vi "test-unscented-kalman-filter-3.vi"() -> (3 "Test good":bool)   [LabVIEW 2019]
uses:
  <vilib>/Analysis/Matrix/Datatypes/RealMatrix.ctl
  <vilib>/Rock Robotics/WPI/ThirdParty/JAS_Junk/TrajLib/MatBuilder_Create.vi
  <vilib>/Rock Robotics/WPI/ThirdParty/JAS_Junk/TrajLib/CallbackHelp_MatrixMinus.vi
  <vilib>/Rock Robotics/WPI/ThirdParty/JAS_Junk/TrajLib/CallbackHelp_MatrixMult_CoerceSizeB.vi
  <vilib>/Rock Robotics/WPI/ThirdParty/JAS_Junk/TrajLib/Trajectory_Library.lvlib
  <vilib>/Analysis/Matrix/NI_Matrix.lvlib
panel:
  out "P Passed":bool
  out "X Passed":bool
  out "P":T1
  out "X":T1
  out "Error":bool
  # "assertTrue(VecBuilder.fill(-0.9, 1, -0.9, 1).isEqual(ret.getFirst(), 1E-5));"
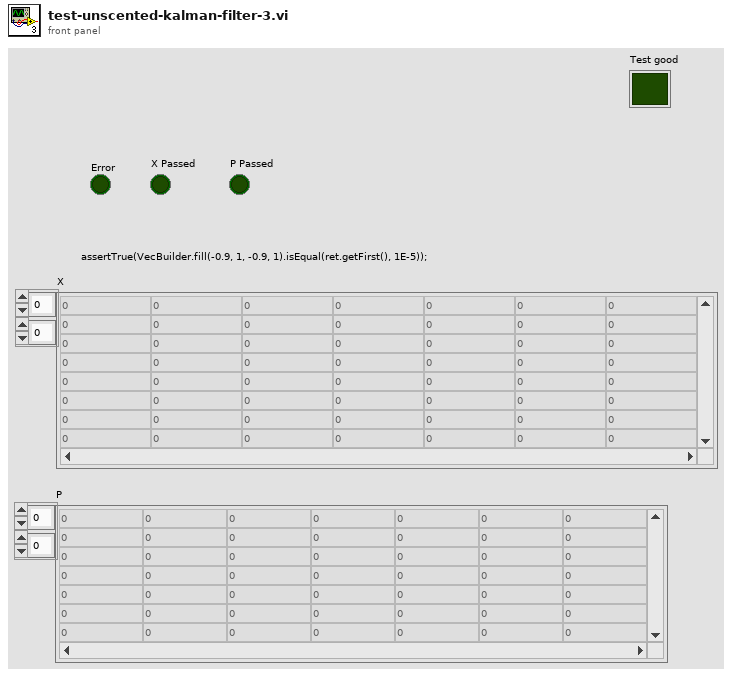
[diagram p1: front panel]
types:
  T1 = typedef "NI_Matrix.lvlib/RealMatrix.ctl" = dbl[][]
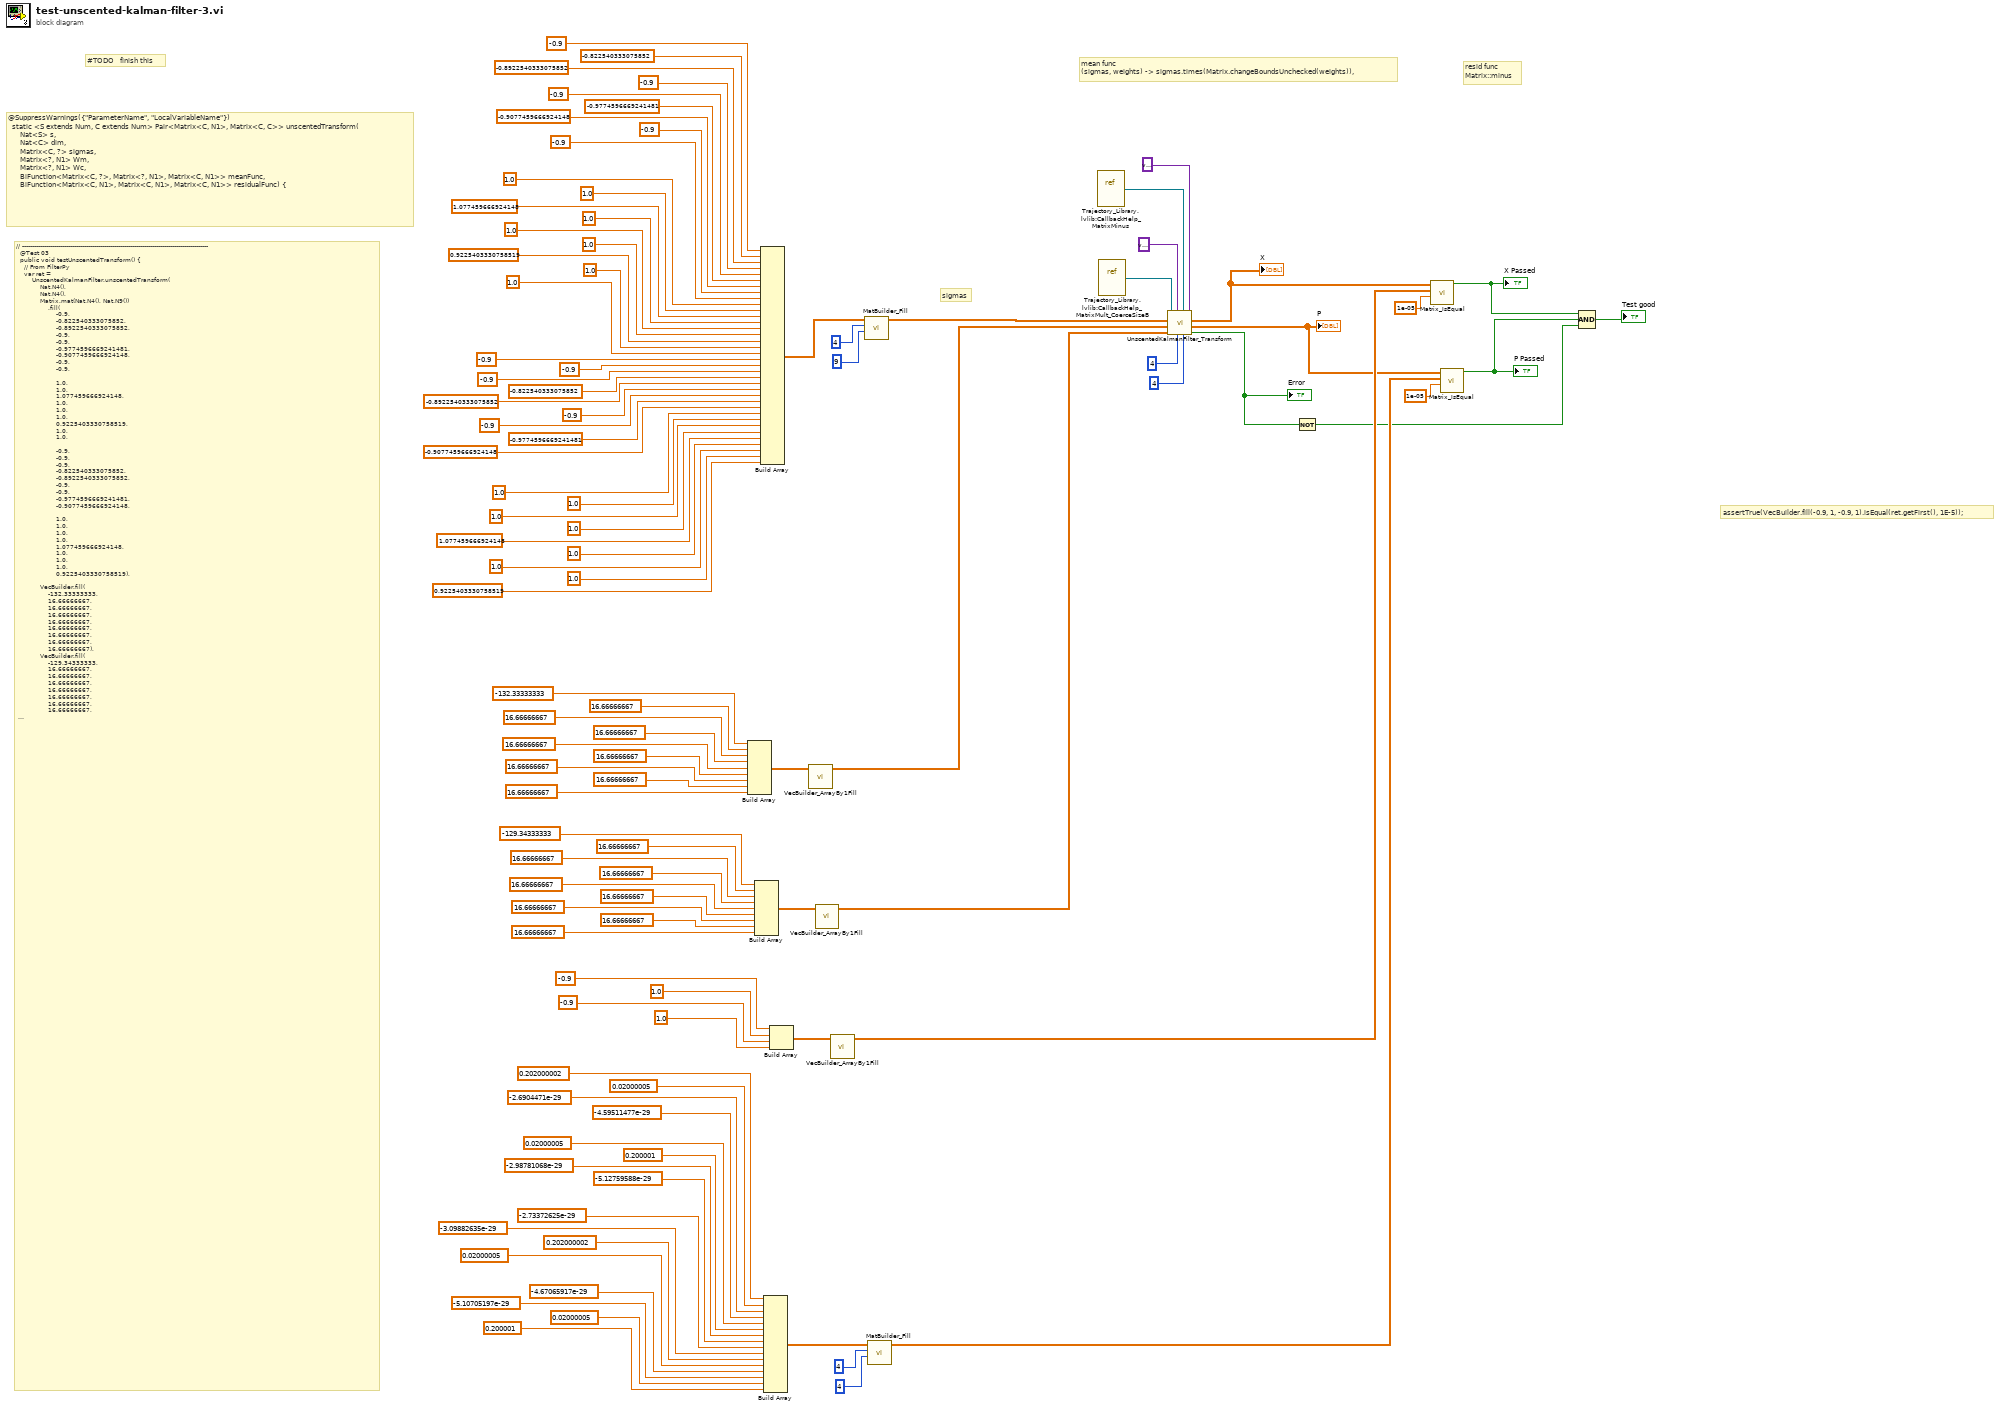
[diagram p0: block diagram]
diagram:
  # "assertTrue(VecBuilder.fill(-0.9, 1, -0.9, 1).isEqual(ret.getFirst(), 1E-5));"
  # "@SuppressWarnings({\"ParameterName\", \"LocalVariableName\"})\n  static <S extends Num, C extends Num> Pair<Matrix<C, N1>, Matrix<C, C>> unscentedTransform(\n      Nat<S> s,\n      Nat<C> dim,\n      Matrix<C, ?> sigmas,\n      Matrix<?, N1> Wm,\n      Matrix<?, N1> Wc,\n      BiFunction<Matrix<C, ?>, Matrix<?, N1>, Matrix<C, N1>> meanFunc,\n      BiFunction<Matrix<C, N1>, Matrix<C, N1>, Matrix<C, N1>> residualFunc) {"
  # "resid func\nMatrix::minus"
  # "mean func\n(sigmas, weights) -> sigmas.times(Matrix.changeBoundsUnchecked(weights)),"
  # "sigmas"
  # "#TODO   finish this"
  # "// ---------------------------------------------------------------------------------------------\n  @Test 03\n  public void testUnscentedTransform() {\n    // From FilterPy\n    var ret =\n        UnscentedKalmanFilter.unscentedTransform(\n            Nat.N4(),\n            Nat.N4(),\n            Matrix.mat(Nat.N4(), Nat.N9())\n                .fill(\n                    -0.9,\n                    -0.822540333075852,\n                    -0.8922540333075852,\n                    -0.9,\n                    -0.9,\n                    -0.9774596669241481,\n                    -0.9077459666924148,\n                    -0.9,\n                    -0.9,\n\n                    1.0,\n                    1.0,\n                    1.077459666924148,\n                    1.0,\n                    1.0,\n                    1.0,\n                    0.9225403330758519,\n                    1.0,\n                    1.0,\n\n                    -0.9,\n                    -0.9,\n                    -0.9,\n                    -0.822540333075852,\n                    -0.8922540333075852,\n                    -0.9,\n                    -0.9,\n                    -0.9774596669241481,\n                    -0.9077459666924148,\n\n                    1.0,\n                    1.0,\n                    1.0,\n                    1.0,\n                    1.077459666924148,\n                    1.0,\n                    1.0,\n                    1.0,\n                    0.9225403330758519),\n\n            VecBuilder.fill(\n                -132.33333333,\n                16.66666667,\n                16.66666667,\n                16.66666667,\n                16.66666667,\n                16.66666667,\n                16.66666667,\n                16.66666667,\n                16.66666667),\n            VecBuilder.fill(\n                -129.34333333,\n                16.66666667,\n                16.66666667,\n                16.66666667,\n                16.66666667,\n                16.66666667,\n                16.66666667,\n                16.66666667,\n                16.66666667),\n\n            (sigmas, weights) -> sigmas.times(Matrix.changeBoundsUnchecked(weights)),\n            Matrix::minus);\n\n    assertTrue(VecBuilder.fill(-0.9, 1, -0.9, 1).isEqual(ret.getFirst(), 1E-5));\n\n    assertTrue(\n        Matrix.mat(Nat.N4(), Nat.N4())\n            .fill(\n                2.02000002e-01,\n                2.00000500e-02,\n                -2.69044710e-29,\n                -4.59511477e-29,\n\n                2.00000500e-02,\n                2.00001000e-01,\n                -2.98781068e-29,\n                -5.12759588e-29,\n\n                -2.73372625e-29,\n                -3.09882635e-29,\n                2.02000002e-01,\n                2.00000500e-02,\n\n                -4.67065917e-29,\n                -5.10705197e-29,\n                2.00000500e-02,\n                2.00001000e-01)\n            .isEqual(ret.getSecond(), 1E-5));\n  }"
  n1 = Build Array(-132.33333333 ("element"), 16.66666667 ("element"), 16.66666667 ("element"), 16.66666667 ("element"), 16.66666667 ("element"), 16.66666667 ("element"), 16.66666667 ("element"), 16.66666667 ("element"), 16.66666667 ("element")) -> (w48:dbl[])
  n2 = Build Array(-129.34333333 ("element"), 16.66666667 ("element"), 16.66666667 ("element"), 16.66666667 ("element"), 16.66666667 ("element"), 16.66666667 ("element"), 16.66666667 ("element"), 16.66666667 ("element"), 16.66666667 ("element")) -> (w38:dbl[])
  n3 = Build Array(-0.9 ("element"), -0.822540333075852 ("element"), -0.8922540333075852 ("element"), -0.9 ("element"), -0.9 ("element"), -0.9774596669241481 ("element"), -0.9077459666924148 ("element"), -0.9 ("element"), -0.9 ("element"), 1.0 ("element"), 1.0 ("element"), 1.077459666924148 ("element"), 1.0 ("element"), 1.0 ("element"), 1.0 ("element"), 0.9225403330758519 ("element"), 1.0 ("element"), 1.0 ("element"), -0.9 ("element"), -0.9 ("element"), -0.9 ("element"), -0.822540333075852 ("element"), -0.8922540333075852 ("element"), -0.9 ("element"), -0.9 ("element"), -0.9774596669241481 ("element"), -0.9077459666924148 ("element"), 1.0 ("element"), 1.0 ("element"), 1.0 ("element"), 1.0 ("element"), 1.077459666924148 ("element"), 1.0 ("element"), 1.0 ("element"), 1.0 ("element"), 0.9225403330758519 ("element")) -> (w101:dbl[])
  n4 = Build Array(0.202000002 ("element"), 0.02000005 ("element"), -2.6904471e-29 ("element"), -4.59511477e-29 ("element"), 0.02000005 ("element"), 0.200001 ("element"), -2.98781068e-29 ("element"), -5.12759588e-29 ("element"), -2.73372625e-29 ("element"), -3.09882635e-29 ("element"), 0.202000002 ("element"), 0.02000005 ("element"), -4.67065917e-29 ("element"), -5.10705197e-29 ("element"), 0.02000005 ("element"), 0.200001 ("element")) -> (w25:dbl[])
  n5 = Build Array(-0.9 ("element"), 1.0 ("element"), -0.9 ("element"), 1.0 ("element")) -> (w31:dbl[])
  n6 = call <vilib>:"VecBuilder_ArrayBy1Fill.vi"("R Array"=w48) -> ("Output Vector"=w37:T1)  [unwired: 10 in]
  n7 = call <vilib>:"VecBuilder_ArrayBy1Fill.vi"("R Array"=w38) -> ("Output Vector"=w36:T1)  [unwired: 10 in]
  n8 = call <vilib>:"VecBuilder_ArrayBy1Fill.vi"("R Array"=w31) -> ("Output Vector"=w29:T1)  [unwired: 10 in]
  n9 = call <vilib>:"MatBuilder_Fill.vi"("Columns"=9, "Rows"=4, "Value List"=w101) -> ("output matrix"=w67:T1)  [unwired: 8 in]
  n10 = call <vilib>:"MatBuilder_Fill.vi"("Columns"=4, "Rows"=4, "Value List"=w25) -> ("output matrix"=w6:T1)  [unwired: 8 in]
  n11 = vi-ref "Trajectory_Library.lvlib:CallbackHelp_MatrixMinus.vi"() -> (w65:refnum<vi>)
  n12 = vi-ref "Trajectory_Library.lvlib:CallbackHelp_MatrixMult_CoerceSizeB.vi"() -> (w64:refnum<vi>)
  n13 = call <vilib>:"UnscentedKalmanFilter_Transform.vi"("ResidualFuncExtra"=variant, "Dim"=4, "residualFunc"=w65, "S"=4, "MeanFuncExtra"=variant, "Wc"=w36, "Wm"=w37, "Sigmas"=w67, "MeanFunc"=w64) -> ("Error"=w5:bool, "P"=w7:T1, "X"=w30:T1)
  "Error" <- w5
  "X" <- w30
  "P" <- w7
  n14 = Not(x=w5) -> (.not. x?=w2:bool)
  n15 = call <vilib>:"Matrix_IsEqual.vi"("Tolerance"=1e-05, "other"=w29, "input matrix"=w30) -> ("Equal"=w4:bool)  [unwired: 8 in]
  "X Passed" <- w4
  n16 = call <vilib>:"Matrix_IsEqual.vi"("Tolerance"=1e-05, "other"=w6, "input matrix"=w7) -> ("Equal"=w3:bool)  [unwired: 8 in]
  "P Passed" <- w3
  n17 = Compound Arithmetic op=AND(w4, w3, w2) -> (→"Test good":bool)
